vi "Control_Verify_Error.vi"(3 "에러 입력(에러 없음)":errorcluster, 4 "timeout (ms)":dbl, 5 "TCP 네트워크 연결 입력":refnum<k5>) -> (0 "에러 출력":errorcluster)   [LabVIEW 2016]
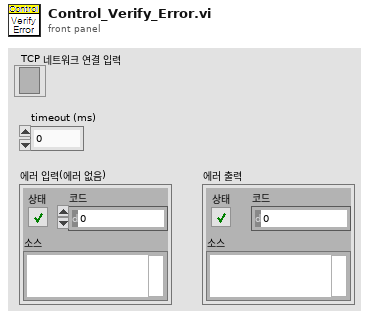
[diagram p1: front panel]
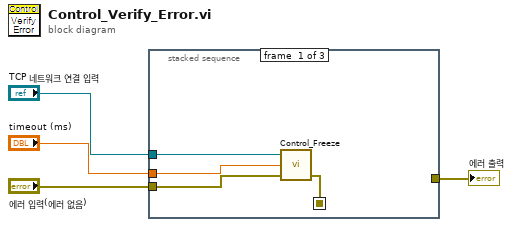
[diagram p0: block diagram]
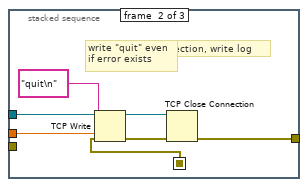
[diagram p2: hidden frame]
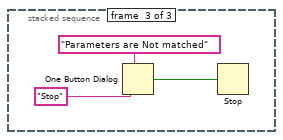
[diagram p3: hidden frame]
diagram:
  n1 = stacked-sequence {
    seq-local: [w5 _ _] -> [_ w10 _]
    tunnel: "TCP 네트워크 연결 입력" -> [w7 w12 _]
    tunnel: "timeout (ms)" -> [w6 w11 _]
    tunnel: "에러 입력(에러 없음)" -> [w8 _ _]
    tunnel: [_ w9 _] -> w4
    frame #0 {
      n2 = call "Control_Freeze.vi"("에러 입력(에러 없음)"=w8, "Timeout (ms)"=w6, "TCP 네트워크 연결 입력"=w7) -> ("에러 출력"=w5:errorcluster)  [unwired: 1 in, 1 out]
    }
    frame #1 {
      # "Close telnet connection, write log"
      # "write \"quit\" even\nif error exists"
      n3 = TCP Write(connection ID=w12, data in="quit\n", error in (no error)=w10, 9:w11) -> (connection ID out=w15:refnum<k5>, error out=w14:errorcluster)  [unwired: 1 out]
      n4 = TCP Close Connection(connection ID=w15, error in (no error)=w14) -> (error out=w9:errorcluster)  [unwired: 1 in, 1 out]
    }
    frame #2 {
      n5 = One Button Dialog(message="Parameters are Not matched" ("메시지"), button name ("OK")="Stop" ("버튼 이름(\"확인\")")) -> (true=w17:bool)
      n6 = Stop(stop? (T)=w17) -> ()
    }
  }
  "에러 출력" <- w4
